vi "Function_for_start record.vi"(0 "Trace names":refnum<vi>, 1 "Start record?":refnum<vi>, 2 "Samples X Signal":u32, 3 "Global Mode":enum32{"Item 0", "Item 1"}(ring), 5 "Refresh \ntime (ms)":i32, 7 "total samples?":refnum<vi>, 9 "status+start record":bool, 11 "error in (no error)":errorcluster, 14 "Class TCP in":T1) -> (4 "Class TCP out":T1, 15 "error out":errorcluster)   [LabVIEW 2022 SP3]
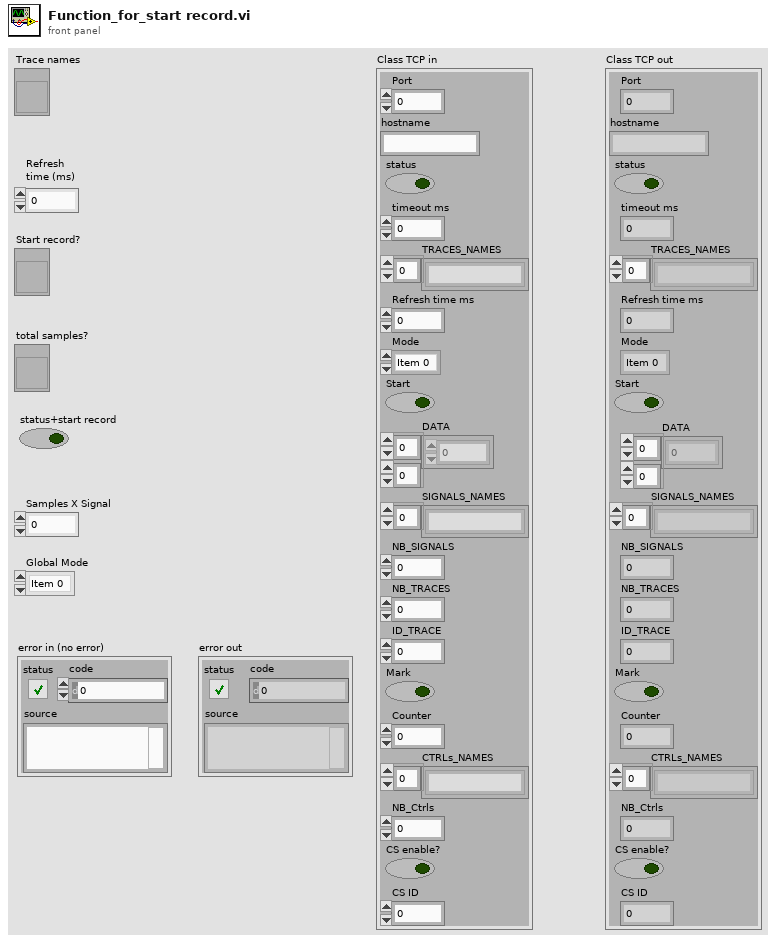
[diagram p1: front panel]
types:
  T1 = cluster{"Port":i32, "hostname":string, "status":bool, "timeout ms":i32, "TRACES_NAMES":string[], "Refresh time ms":i32, "Mode":enum32{"Item 0", "Item 1"}, "Start":bool, "DATA":sgl[][], "SIGNALS_NAMES":string[], "NB_SIGNALS":i32, "NB_TRACES":i32, "ID_TRACE":i32, "Mark":bool, "Counter":i32, "CTRLs_NAMES":string[], "NB_Ctrls":i32, "CS enable?":bool, "CS ID":i32}
  T2 = cluster{"TRACE_SIZE":i32, "CS_ID":i32, "TRACE ID":i32, "CMD":i32, "DATA(M)":i32}
  T3 = cluster{"timeout ms":i32, "remote port":u16, "Address":string}
  T4 = cluster{"SIZE":i32, " TRACE DATA":sgl[], "TRACE_SIZE":i32, "NB_TRACES":i32, "NB_TRACED_SIGNALS":i32, "NAMES TRACED SIGNALS":string[], "NAMES TRACES":string[], "CS STATUS":i32, "NB_CSs":i32, "NAMES CSs":string[], "DATA (M)":sgl[], "CMD":i32}
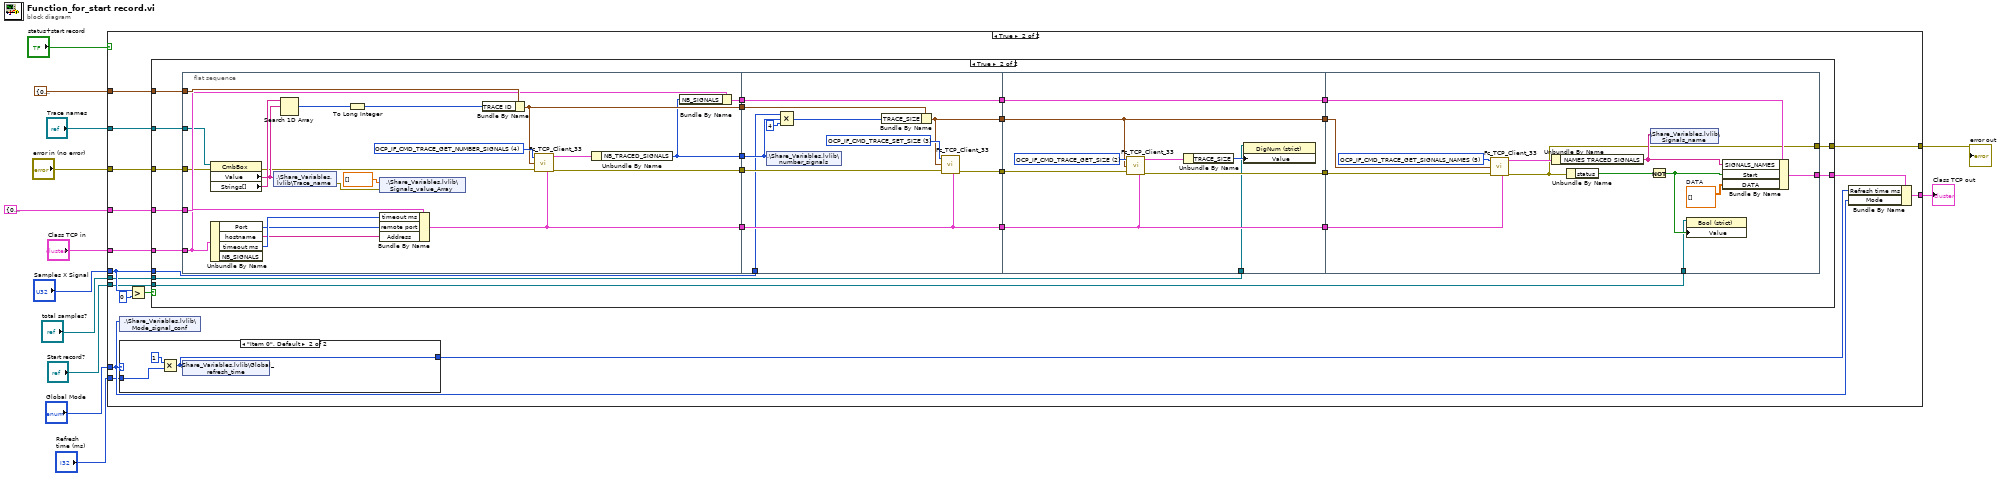
[diagram p0: block diagram]
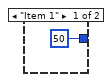
[diagram p4: hidden frame]
diagram:
  n1 = case shown="True" "status+start record" {
    tunnel: "Class TCP in" -> [w15 w27]
    tunnel: [w15 w31] -> w8
    tunnel: T3 {"timeout ms"=0, "remote port"=0, "Address"=""} ("Comunication Cluster") -> [_ w25]
    tunnel: T2 {"TRACE_SIZE"=0, "CS_ID"=0, "TRACE ID"=0, "CMD"=0, "DATA(M)"=0} ("Input Cluster") -> [_ w24]
    tunnel: "Samples X Signal" -> [_ w23]
    tunnel: "Global Mode" -> [_ w22]
    tunnel: "Refresh \ntime (ms)" -> [_ w21]
    tunnel: "Trace names" -> [_ w20]
    tunnel: "Start record?" -> [_ w19]
    tunnel: "total samples?" -> [_ w18]
    tunnel: [w14 w17] -> w2
    tunnel: "error in (no error)" -> [w14 w16]
    frame False {
    }
    frame True {
      n2 = shared-variable ".\\Share_Variables.lvlib\\Mode_signal_conf"(w22) -> ()  [unwired: 1 in, 1 out]
      n3 = case shown="\"Item 0\", Default" w22 {
        tunnel: [50 ("Refresh time (sec)") w114] -> w30
        tunnel: w21 -> [_ w113]
        frame "Item 1" {
        }
        frame "Item 0", Default {
          n4 = Multiply(x=1, y=w113) -> (x*y=w114:i32)
          n5 = shared-variable ".\\Share_Variables.lvlib\\Global_refresh_time"(w114) -> ()  [unwired: 1 in, 1 out]
        }
      }
      n6 = Greater?(x=w23, y=0) -> (0:w29:bool)
      n7 = case shown="True" w29 {
        tunnel: w27 -> [w33 w56]
        tunnel: [w33 w55] -> w26
        tunnel: w25 -> [_ w54]
        tunnel: w24 -> [_ w53]
        tunnel: w23 -> [_ w40]
        tunnel: w20 -> [_ w38]
        tunnel: w19 -> [_ w37]
        tunnel: w18 -> [_ w36]
        tunnel: [w32 w35] -> w17
        tunnel: w16 -> [w32 w34]
        frame False {
        }
        frame True {
          n8 = flat-sequence {
            tunnel: w56 -> [w62]
            tunnel: [w75] -> w52
            tunnel: [w61] -> w50
            tunnel: [w69] -> w48
            tunnel: [w64] -> w47
            tunnel: w54 -> [w68]
            tunnel: w53 -> [w67]
            tunnel: [w60] -> w45
            tunnel: w38 -> [w58]
            tunnel: w34 -> [w57]
            tunnel: w52 -> [w88]
            tunnel: [w87] -> w51
            tunnel: w50 -> [w89]
            tunnel: [w89] -> w49
            tunnel: w48 -> [w84]
            tunnel: w47 -> [w85]
            tunnel: [w85] -> w46
            tunnel: w45 -> [w83]
            tunnel: w40 -> [w80]
            tunnel: [w79] -> w39
            tunnel: w51 -> [w97]
            tunnel: [w96] -> w44
            tunnel: w49 -> [w98]
            tunnel: [w98] -> w43
            tunnel: [w94] -> w42
            tunnel: w46 -> [w91]
            tunnel: [w91] -> w41
            tunnel: w39 -> [w94]
            tunnel: w36 -> [w90]
            tunnel: w43 -> [w111]
            tunnel: [w110] -> w55
            tunnel: w44 -> [w108]
            tunnel: w41 -> [w106]
            tunnel: w42 -> [w105]
            tunnel: w37 -> [w100]
            tunnel: [w99] -> w35
            frame #0 {
              w74 = 4 items=["OCP_IF_CMD_TRACE_READ", "OCP_IF_CMD_TRACE_RESET", "OCP_IF_CMD_TRACE_GET_SIZE", "OCP_IF_CMD_TRACE_SET_SIZE", "OCP_IF_CMD_TRACE_GET_NUMBER_SIGNALS", "OCP_IF_CMD_TRACE_GET_SIGNALS_NAMES", "OCP_IF_CMD_TRACE_GET_NUMBER_TRACES", "OCP_IF_CMD_TRACE_GET_TRACES_NAMES", "OCP_IF_CMD_TRACE_GET_ADDRESS", "OCP_IF_CMD_CS_STATUS", "OCP_IF_CMD_CS_ENABLE", "OCP_IF_CMD_CS_DISABLE", "OCP_IF_CMD_CS_CONTROLLER_IF", "OCP_IF_CMD_CS_HARDWARE_IF", "OCP_IF_CMD_CS_GET_NUMBER_CONTROLLERS", "OCP_IF_CMD_CS_GET_CONTROLLERS_NAMES", "OCP_IF_CMD_PLATFORM_ID", "OCP_IF_CMD_PLATFORM_IF", "OCP_IF_CMD_OPIL_UPDATE_MEASUREMENTS", "OCP_IF_CMD_OPIL_UPDATE_SIM_DATA", "OCP_IF_CMD_OPIL_RUN_CONTROL", "OCP_IF_CMD_OPIL_INITIALIZE_CONTROL", "OCP_IF_CMD_OPIL_GET_CONTROL", "OCP_IF_CMD_OPIL_GET_CONTROLLER_DATA", "OCP_IF_CMD_END"] ("CMD")
              n9 = Unbundle By Name(w62) -> ("Port"=w72:i32, "hostname"=w71:string, "timeout ms"=w73:i32)  [unwired: 1 out]
              n10 = property on="Property Node" class="CmbBox"(reference=w58, error in=w57) -> (error out=w70:errorcluster, "Value"=w76:string, "Strings[]"=w78:string[])  [unwired: 1 out]
              n11 = shared-variable ".\\Share_Variables.lvlib\\Trace_name"(w76) -> (error out=w66:errorcluster)  [unwired: 1 in]
              n12 = Search 1D Array(1D array=w78, element=w76) -> (index of element=w77:i32)  [unwired: 1 in]
              n13 = To Long Integer(number=w77) -> (32bit integer=w59:i32)
              n14 = shared-variable ".\\Share_Variables.lvlib\\Signals_value_Array"(dbl[] [] ("Signals_value_Array"), error in=w66) -> ()  [unwired: 1 out]
              n15 = Bundle By Name(cluster=w68, "timeout ms"=w73, "remote port"=w72, "Address"=w71) -> (w64:T3)
              n16 = Bundle By Name(cluster=w67, "TRACE ID"=w59) -> (w69:T2)
              n17 = call "Fc_TCP_Client_33.vi"("CMD"=w74, "Input Cluster"=w69, "error in (no error)"=w70, "Comunication Cluster"=w64) -> ("Output cluster"=w63:T4, "error out"=w75:errorcluster)  [unwired: 4 in, 1 out]
              n18 = Unbundle By Name(w63) -> ("NB_TRACED_SIGNALS"=w60:i32)
              n19 = Bundle By Name(cluster=w62, "NB_SIGNALS"=w60) -> (w61:T1)
            }
            frame #1 {
              w86 = 3 items=["OCP_IF_CMD_TRACE_READ", "OCP_IF_CMD_TRACE_RESET", "OCP_IF_CMD_TRACE_GET_SIZE", "OCP_IF_CMD_TRACE_SET_SIZE", "OCP_IF_CMD_TRACE_GET_NUMBER_SIGNALS", "OCP_IF_CMD_TRACE_GET_SIGNALS_NAMES", "OCP_IF_CMD_TRACE_GET_NUMBER_TRACES", "OCP_IF_CMD_TRACE_GET_TRACES_NAMES", "OCP_IF_CMD_TRACE_GET_ADDRESS", "OCP_IF_CMD_CS_STATUS", "OCP_IF_CMD_CS_ENABLE", "OCP_IF_CMD_CS_DISABLE", "OCP_IF_CMD_CS_CONTROLLER_IF", "OCP_IF_CMD_CS_HARDWARE_IF", "OCP_IF_CMD_CS_GET_NUMBER_CONTROLLERS", "OCP_IF_CMD_CS_GET_CONTROLLERS_NAMES", "OCP_IF_CMD_PLATFORM_ID", "OCP_IF_CMD_PLATFORM_IF", "OCP_IF_CMD_OPIL_UPDATE_MEASUREMENTS", "OCP_IF_CMD_OPIL_UPDATE_SIM_DATA", "OCP_IF_CMD_OPIL_RUN_CONTROL", "OCP_IF_CMD_OPIL_INITIALIZE_CONTROL", "OCP_IF_CMD_OPIL_GET_CONTROL", "OCP_IF_CMD_OPIL_GET_CONTROLLER_DATA", "OCP_IF_CMD_END"] ("CMD")
              n20 = shared-variable ".\\Share_Variables.lvlib\\number_signals"(w83) -> ()  [unwired: 1 in, 1 out]
              n21 = Compound Arithmetic op=MULTIPLY(w80, w83, 4 ("value")) -> (w81:u32)
              n22 = Bundle By Name(cluster=w84, "TRACE_SIZE"=w81) -> (w79:T2)
              n23 = call "Fc_TCP_Client_33.vi"("CMD"=w86, "Input Cluster"=w79, "error in (no error)"=w88, "Comunication Cluster"=w85) -> ("error out"=w87:errorcluster)  [unwired: 4 in, 2 out]
            }
            frame #2 {
              w95 = 2 items=["OCP_IF_CMD_TRACE_READ", "OCP_IF_CMD_TRACE_RESET", "OCP_IF_CMD_TRACE_GET_SIZE", "OCP_IF_CMD_TRACE_SET_SIZE", "OCP_IF_CMD_TRACE_GET_NUMBER_SIGNALS", "OCP_IF_CMD_TRACE_GET_SIGNALS_NAMES", "OCP_IF_CMD_TRACE_GET_NUMBER_TRACES", "OCP_IF_CMD_TRACE_GET_TRACES_NAMES", "OCP_IF_CMD_TRACE_GET_ADDRESS", "OCP_IF_CMD_CS_STATUS", "OCP_IF_CMD_CS_ENABLE", "OCP_IF_CMD_CS_DISABLE", "OCP_IF_CMD_CS_CONTROLLER_IF", "OCP_IF_CMD_CS_HARDWARE_IF", "OCP_IF_CMD_CS_GET_NUMBER_CONTROLLERS", "OCP_IF_CMD_CS_GET_CONTROLLERS_NAMES", "OCP_IF_CMD_PLATFORM_ID", "OCP_IF_CMD_PLATFORM_IF", "OCP_IF_CMD_OPIL_UPDATE_MEASUREMENTS", "OCP_IF_CMD_OPIL_UPDATE_SIM_DATA", "OCP_IF_CMD_OPIL_RUN_CONTROL", "OCP_IF_CMD_OPIL_INITIALIZE_CONTROL", "OCP_IF_CMD_OPIL_GET_CONTROL", "OCP_IF_CMD_OPIL_GET_CONTROLLER_DATA", "OCP_IF_CMD_END"] ("CMD")
              n24 = call "Fc_TCP_Client_33.vi"("CMD"=w95, "Input Cluster"=w94, "error in (no error)"=w97, "Comunication Cluster"=w91) -> ("Output cluster"=w93:T4, "error out"=w96:errorcluster)  [unwired: 4 in, 1 out]
              n25 = Unbundle By Name(w93) -> ("TRACE_SIZE"=w92:i32)
              n26 = property on="Property Node" class="DigNum (strict)"(reference=w90, "Value"=w92) -> ()  [unwired: 1 in, 2 out]
            }
            frame #3 {
              w101 = sgl[][] []  # DATA
              w107 = 5 items=["OCP_IF_CMD_TRACE_READ", "OCP_IF_CMD_TRACE_RESET", "OCP_IF_CMD_TRACE_GET_SIZE", "OCP_IF_CMD_TRACE_SET_SIZE", "OCP_IF_CMD_TRACE_GET_NUMBER_SIGNALS", "OCP_IF_CMD_TRACE_GET_SIGNALS_NAMES", "OCP_IF_CMD_TRACE_GET_NUMBER_TRACES", "OCP_IF_CMD_TRACE_GET_TRACES_NAMES", "OCP_IF_CMD_TRACE_GET_ADDRESS", "OCP_IF_CMD_CS_STATUS", "OCP_IF_CMD_CS_ENABLE", "OCP_IF_CMD_CS_DISABLE", "OCP_IF_CMD_CS_CONTROLLER_IF", "OCP_IF_CMD_CS_HARDWARE_IF", "OCP_IF_CMD_CS_GET_NUMBER_CONTROLLERS", "OCP_IF_CMD_CS_GET_CONTROLLERS_NAMES", "OCP_IF_CMD_PLATFORM_ID", "OCP_IF_CMD_PLATFORM_IF", "OCP_IF_CMD_OPIL_UPDATE_MEASUREMENTS", "OCP_IF_CMD_OPIL_UPDATE_SIM_DATA", "OCP_IF_CMD_OPIL_RUN_CONTROL", "OCP_IF_CMD_OPIL_INITIALIZE_CONTROL", "OCP_IF_CMD_OPIL_GET_CONTROL", "OCP_IF_CMD_OPIL_GET_CONTROLLER_DATA", "OCP_IF_CMD_END"] ("CMD")
              n27 = call "Fc_TCP_Client_33.vi"("CMD"=w107, "Input Cluster"=w105, "error in (no error)"=w108, "Comunication Cluster"=w106) -> ("Output cluster"=w109:T4, "error out"=w99:errorcluster)  [unwired: 4 in, 1 out]
              n28 = Unbundle By Name(w109) -> ("NAMES TRACED SIGNALS"=w103:string[])
              n29 = Unbundle By Name(w99) -> ("status"=w104:bool)
              n30 = Not(x=w104) -> (.not. x?=w102:bool)
              n31 = shared-variable ".\\Share_Variables.lvlib\\Signals_name"(w103) -> ()  [unwired: 1 in, 1 out]
              n32 = property class="Bool (strict)"(reference=w100, "Value"=w102) -> ()  [unwired: 1 in, 2 out]
              n33 = Bundle By Name(cluster=w111, "SIGNALS_NAMES"=w103, "Start"=w102, "DATA"=w101) -> (w110:T1)
            }
          }
        }
      }
      n34 = Bundle By Name(cluster=w26, "Refresh time ms"=w30, "Mode"=w22) -> (w31:T1)
    }
  }
  "Class TCP out" <- w8
  "error out" <- w2
